vi "例5.11  “按名称打包（捆绑）”函数.vi"() -> ()   [LabVIEW 2017]
panel:
  out "簇":cluster{string, i32, bool}={"ABC", 1, FALSE}
  out "输出簇":cluster{string, i32, bool}
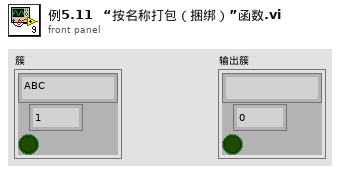
[diagram p1: front panel]
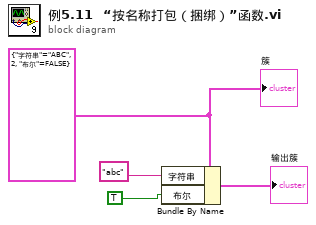
[diagram p0: block diagram]
diagram:
  w4 = cluster{"字符串":string, i32, "布尔":bool} {"字符串"="ABC", 2, "布尔"=FALSE}
  n1 = Bundle By Name(cluster=w4, "字符串"="abc", "布尔"=TRUE) -> (→"输出簇":cluster{"字符串":string, i32, "布尔":bool})
  "簇" <- w4
